vi "ProtocolAnalysis 2.vi"(7 "Braodcast_Data":string, 8 "error in":errorcluster caption="错误输入", 11 "IP":refnum<k5>) -> (0 "error out":errorcluster caption="错误输出", 1 "Disconnected":bool, 3 "IP 2":refnum<k5>)   [LabVIEW 2015]
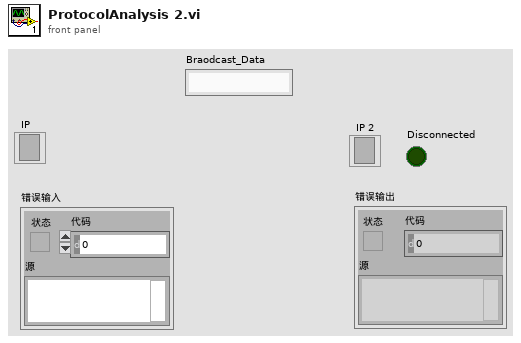
[diagram p1: front panel]
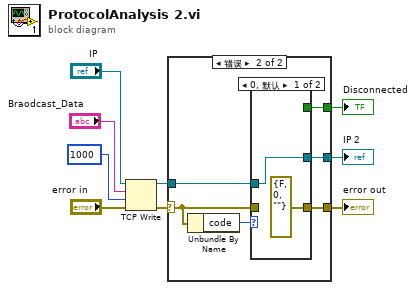
[diagram p0: block diagram]
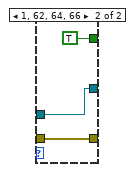
[diagram p3: hidden frame]
diagram:
  n1 = TCP Write(connection ID="IP", data in="Braodcast_Data", error in (no error)="error in", 9:1000 ("timeout ms (25000)")) -> (connection ID out=w2:refnum<k5>, error out=w1:errorcluster)  [unwired: 1 out]
  n2 = case shown="错误" w1 {
    selector: w1 -> [w11 w16]
    tunnel: [w11 w15] -> w5
    tunnel: w2 -> [w10 w14]
    tunnel: [w10 w13] -> w8
    tunnel: [_ w12] -> w7
    frame No Error {
    }
    frame Error {
      n3 = Unbundle By Name(w16) -> ("code"=w17:i32)
      n4 = case shown="0, 默认" w17 {
        tunnel: w16 -> [_ w20]
        tunnel: [errorcluster {"status"=FALSE, "code"=0, "source"=""} ("error IO") w20] -> w15
        tunnel: w14 -> [w19 w21]
        tunnel: [w19 w21] -> w13
        tunnel: [_ TRUE] -> w12
        frame 0, Default {
        }
        frame 1, 62, 64, 66 {
        }
      }
    }
  }
  "error out" <- w5
  "IP 2" <- w8
  "Disconnected" <- w7
